vi "Visible_Ch _11-20.vi"(8 "Unit PN":string) -> ()   [LabVIEW 2017]
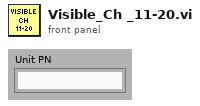
[diagram p1: front panel]
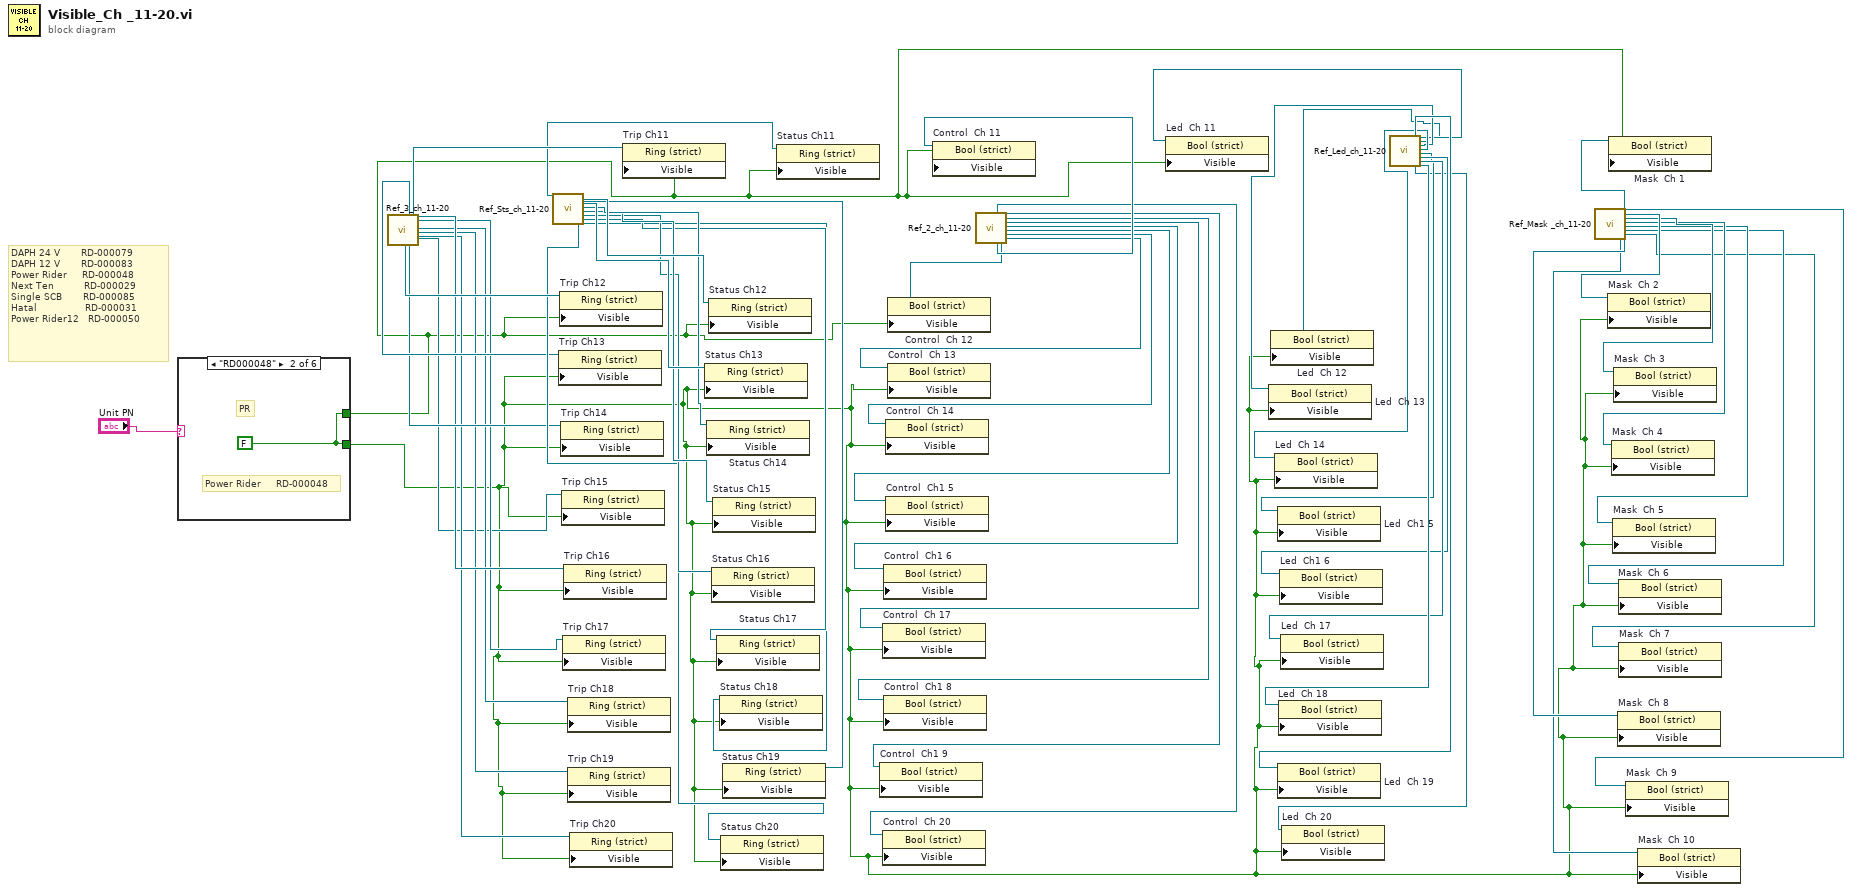
[diagram p0: block diagram]
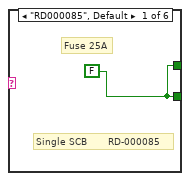
[diagram p2: hidden frame]
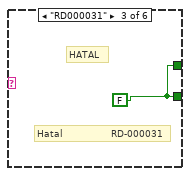
[diagram p3: hidden frame]
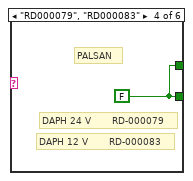
[diagram p4: hidden frame]
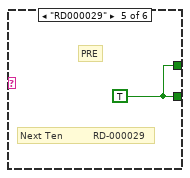
[diagram p5: hidden frame]
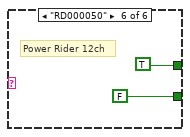
[diagram p6: hidden frame]
diagram:
  # "DAPH 24 V  \t    RD-000079\nDAPH 12 V  \t    RD-000083\nPower Rider \t   RD-000048\nNext Ten  \t       RD-000029\nSingle SCB       RD-000085 \nHatal                RD-000031\nPower Rider12   RD-000050"
  n1 = case shown="\"RD000048\"" "Unit PN" {
    tunnel: [w54 w55 w56 w57 w58 FALSE] -> w2
    tunnel: [w54 w55 w56 w57 w58 TRUE] -> w1
    frame "RD000085", Default {
      w54 = FALSE
      # "Single SCB       RD-000085"
      # "Fuse 25A"
    }
    frame "RD000048" {
      w55 = FALSE
      # "Power Rider \t   RD-000048"
      # "PR"
    }
    frame "RD000031" {
      w56 = FALSE
      # "Hatal                RD-000031"
      # "HATAL"
    }
    frame "RD000079", "RD000083" {
      w57 = FALSE
      # "DAPH 12 V  \t    RD-000083"
      # "DAPH 24 V  \t    RD-000079"
      # "PALSAN"
    }
    frame "RD000029" {
      w58 = TRUE
      # "Next Ten  \t       RD-000029"
      # "PRE"
    }
    frame "RD000050" {
      # "Power Rider 12ch"
    }
  }
  n2 = call "Ref_3_ch_11-20.vi"() -> ("Trip  Ch 11 out"=w53:refnum<vi>, "Trip  Ch 12 out"=w50:refnum<vi>, "Trip  Ch 13 out"=w34:refnum<vi>, "Trip  Ch 14 out"=w33:refnum<vi>, "Trip  Ch 15 out"=w14:refnum<vi>, "Trip  Ch 16 out"=w32:refnum<vi>, "Trip  Ch 17 out"=w31:refnum<vi>, "Trip  Ch 18 out"=w30:refnum<vi>, "Trip  Ch 19 out"=w29:refnum<vi>, "Trip  Ch 20 out"=w28:refnum<vi>)  [unwired: 18 in]
  n3 = call "Ref_Sts_ch_11-20.vi"() -> ("Status Ch 19 out"=w36:refnum<vi>, "Status Ch 20 out"=w35:refnum<vi>, "Status Ch 11 out"=w52:refnum<vi>, "Status Ch 12 out"=w42:refnum<vi>, "Status Ch 13 out"=w41:refnum<vi>, "Status Ch 14 out"=w40:refnum<vi>, "Status Ch 15 out"=w39:refnum<vi>, "Status Ch 16 out"=w38:refnum<vi>, "Status Ch 17 out"=w37:refnum<vi>, "Status Ch 18 out"=w25:refnum<vi>)  [unwired: 18 in]
  n4 = property on="Trip Ch13" class="Ring (strict)"(reference=w34, "Visible"=w2) -> ()  [unwired: 1 in, 2 out]
  n5 = property on="Trip Ch12" class="Ring (strict)"(reference=w50, "Visible"=w1) -> ()  [unwired: 1 in, 2 out]
  n6 = property on="Trip Ch14" class="Ring (strict)"(reference=w33, "Visible"=w2) -> ()  [unwired: 1 in, 2 out]
  n7 = property on="Trip Ch15" class="Ring (strict)"(reference=w14, "Visible"=w2) -> ()  [unwired: 1 in, 2 out]
  n8 = property on="Trip Ch17" class="Ring (strict)"(reference=w31, "Visible"=w2) -> ()  [unwired: 1 in, 2 out]
  n9 = property on="Trip Ch16" class="Ring (strict)"(reference=w32, "Visible"=w2) -> ()  [unwired: 1 in, 2 out]
  n10 = property on="Trip Ch18" class="Ring (strict)"(reference=w30, "Visible"=w2) -> ()  [unwired: 1 in, 2 out]
  n11 = property on="Trip Ch19" class="Ring (strict)"(reference=w29, "Visible"=w2) -> ()  [unwired: 1 in, 2 out]
  n12 = property on="Trip Ch20" class="Ring (strict)"(reference=w28, "Visible"=w2) -> ()  [unwired: 1 in, 2 out]
  n13 = property on="Trip Ch11" class="Ring (strict)"(reference=w53, "Visible"=w1) -> ()  [unwired: 1 in, 2 out]
  n14 = property on="Status Ch13" class="Ring (strict)"(reference=w41, "Visible"=w2) -> ()  [unwired: 1 in, 2 out]
  n15 = property on="Status Ch14" class="Ring (strict)"(reference=w40, "Visible"=w2) -> ()  [unwired: 1 in, 2 out]
  n16 = property on="Status Ch12" class="Ring (strict)"(reference=w42, "Visible"=w1) -> ()  [unwired: 1 in, 2 out]
  n17 = property on="Status Ch16" class="Ring (strict)"(reference=w38, "Visible"=w2) -> ()  [unwired: 1 in, 2 out]
  n18 = property on="Status Ch15" class="Ring (strict)"(reference=w39, "Visible"=w2) -> ()  [unwired: 1 in, 2 out]
  n19 = property on="Status Ch17" class="Ring (strict)"(reference=w37, "Visible"=w2) -> ()  [unwired: 1 in, 2 out]
  n20 = property on="Status Ch18" class="Ring (strict)"(reference=w25, "Visible"=w2) -> ()  [unwired: 1 in, 2 out]
  n21 = property on="Status Ch20" class="Ring (strict)"(reference=w35, "Visible"=w2) -> ()  [unwired: 1 in, 2 out]
  n22 = property on="Status Ch19" class="Ring (strict)"(reference=w36, "Visible"=w2) -> ()  [unwired: 1 in, 2 out]
  n23 = property on="Status Ch11" class="Ring (strict)"(reference=w52, "Visible"=w1) -> ()  [unwired: 1 in, 2 out]
  n24 = call "Ref_2_ch_11-20.vi"() -> ("Control  Ch 20 out"=w43:refnum<vi>, "Control  Ch 11 out"=w51:refnum<vi>, "Control  Ch 19 out"=w44:refnum<vi>, "Control  Ch 12 out"=w49:refnum<vi>, "Control  Ch 18 out"=w45:refnum<vi>, "Control  Ch 17 out"=w46:refnum<vi>, "Control  Ch 16 out"=w26:refnum<vi>, "Control  Ch 15 out"=w47:refnum<vi>, "Control  Ch 14 out"=w48:refnum<vi>, "Control  Ch 13 out"=w27:refnum<vi>)  [unwired: 17 in, 1 out]
  n25 = property on="Control  Ch1 9" class="Bool (strict)"(reference=w44, "Visible"=w2) -> ()  [unwired: 1 in, 2 out]
  n26 = property on="Control  Ch 17" class="Bool (strict)"(reference=w46, "Visible"=w2) -> ()  [unwired: 1 in, 2 out]
  n27 = property on="Control  Ch 20" class="Bool (strict)"(reference=w43, "Visible"=w2) -> ()  [unwired: 1 in, 2 out]
  n28 = property on="Control  Ch1 6" class="Bool (strict)"(reference=w26, "Visible"=w2) -> ()  [unwired: 1 in, 2 out]
  n29 = property on="Control  Ch1 8" class="Bool (strict)"(reference=w45, "Visible"=w2) -> ()  [unwired: 1 in, 2 out]
  n30 = property on="Control  Ch 14" class="Bool (strict)"(reference=w48, "Visible"=w2) -> ()  [unwired: 1 in, 2 out]
  n31 = property on="Control  Ch1 5" class="Bool (strict)"(reference=w47, "Visible"=w2) -> ()  [unwired: 1 in, 2 out]
  n32 = property on="Control  Ch 12" class="Bool (strict)"(reference=w49, "Visible"=w1) -> ()  [unwired: 1 in, 2 out]
  n33 = property on="Control  Ch 13" class="Bool (strict)"(reference=w27, "Visible"=w2) -> ()  [unwired: 1 in, 2 out]
  n34 = property on="Control  Ch 11" class="Bool (strict)"(reference=w51, "Visible"=w1) -> ()  [unwired: 1 in, 2 out]
  n35 = call "Ref_Led_ch_11-20.vi"() -> ("Led Ch 19 out"=w24:refnum<vi>, "Led Ch 20 out"=w17:refnum<vi>, "Led Ch 11 out"=w16:refnum<vi>, "Led Ch 12 out"=w15:refnum<vi>, "Led Ch 13 out"=w18:refnum<vi>, "Led Ch 14 out"=w19:refnum<vi>, "Led Ch 15 out"=w20:refnum<vi>, "Led Ch 16 out"=w21:refnum<vi>, "Led Ch 17 out"=w22:refnum<vi>, "Led Ch 18 out"=w23:refnum<vi>)  [unwired: 18 in]
  n36 = property on="Led  Ch 11" class="Bool (strict)"(reference=w16, "Visible"=w1) -> ()  [unwired: 1 in, 2 out]
  n37 = property on="Led  Ch 13" class="Bool (strict)"(reference=w18, "Visible"=w2) -> ()  [unwired: 1 in, 2 out]
  n38 = property on="Led  Ch 12" class="Bool (strict)"(reference=w15, "Visible"=w2) -> ()  [unwired: 1 in, 2 out]
  n39 = property on="Led  Ch 14" class="Bool (strict)"(reference=w19, "Visible"=w2) -> ()  [unwired: 1 in, 2 out]
  n40 = property on="Led  Ch1 5" class="Bool (strict)"(reference=w20, "Visible"=w2) -> ()  [unwired: 1 in, 2 out]
  n41 = property on="Led  Ch 19" class="Bool (strict)"(reference=w24, "Visible"=w2) -> ()  [unwired: 1 in, 2 out]
  n42 = property on="Led  Ch 18" class="Bool (strict)"(reference=w23, "Visible"=w2) -> ()  [unwired: 1 in, 2 out]
  n43 = property on="Led  Ch1 6" class="Bool (strict)"(reference=w21, "Visible"=w2) -> ()  [unwired: 1 in, 2 out]
  n44 = property on="Led  Ch 17" class="Bool (strict)"(reference=w22, "Visible"=w2) -> ()  [unwired: 1 in, 2 out]
  n45 = property on="Led  Ch 20" class="Bool (strict)"(reference=w17, "Visible"=w2) -> ()  [unwired: 1 in, 2 out]
  n46 = call "Ref_Mask _ch_11-20.vi"() -> ("Mask Ch 19 out"=w4:refnum<vi>, "Mask Ch 20 out"=w6:refnum<vi>, "Mask Ch 11 out"=w5:refnum<vi>, "Mask Ch 12 out"=w13:refnum<vi>, "Mask Ch 13 out"=w12:refnum<vi>, "Mask Ch 14 out"=w11:refnum<vi>, "Mask Ch 15 out"=w10:refnum<vi>, "Mask Ch 16 out"=w9:refnum<vi>, "Mask Ch 17 out"=w8:refnum<vi>, "Mask Ch 18 out"=w7:refnum<vi>)  [unwired: 18 in]
  n47 = property on="Mask  Ch 2" class="Bool (strict)"(reference=w13, "Visible"=w2) -> ()  [unwired: 1 in, 2 out]
  n48 = property on="Mask  Ch 1" class="Bool (strict)"(reference=w5, "Visible"=w1) -> ()  [unwired: 1 in, 2 out]
  n49 = property on="Mask  Ch 4" class="Bool (strict)"(reference=w11, "Visible"=w2) -> ()  [unwired: 1 in, 2 out]
  n50 = property on="Mask  Ch 5" class="Bool (strict)"(reference=w10, "Visible"=w2) -> ()  [unwired: 1 in, 2 out]
  n51 = property on="Mask  Ch 3" class="Bool (strict)"(reference=w12, "Visible"=w2) -> ()  [unwired: 1 in, 2 out]
  n52 = property on="Mask  Ch 8" class="Bool (strict)"(reference=w7, "Visible"=w2) -> ()  [unwired: 1 in, 2 out]
  n53 = property on="Mask  Ch 6" class="Bool (strict)"(reference=w9, "Visible"=w2) -> ()  [unwired: 1 in, 2 out]
  n54 = property on="Mask  Ch 7" class="Bool (strict)"(reference=w8, "Visible"=w2) -> ()  [unwired: 1 in, 2 out]
  n55 = property on="Mask  Ch 9" class="Bool (strict)"(reference=w4, "Visible"=w2) -> ()  [unwired: 1 in, 2 out]
  n56 = property on="Mask  Ch 10" class="Bool (strict)"(reference=w6, "Visible"=w2) -> ()  [unwired: 1 in, 2 out]
